vi "Maquina01Refrescos_1.vi"() -> ()   [LabVIEW 2018]
uses:
  EdoMaq1Refrescos.ctl
panel:
  in  "stop 2":bool
  out "Elapsed Time (s)":dbl
  out "Cambio":i32
  out "Suma":i32
  out "Edo":T1
  in  "stop":bool
  in  "Cancel Button":bool
  in  "$10":bool
  in  "$5":bool
  in  "$1":bool
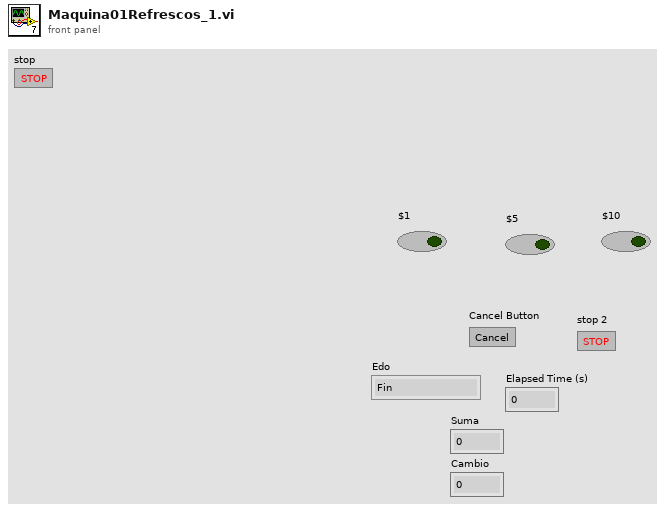
[diagram p1: front panel]
types:
  T1 = typedef "EdoMaq1Refrescos.ctl" = enum16{"Fin", "Espera", "JuntaDinero", "Entrega", "RegresaCambio", "Cancela"}
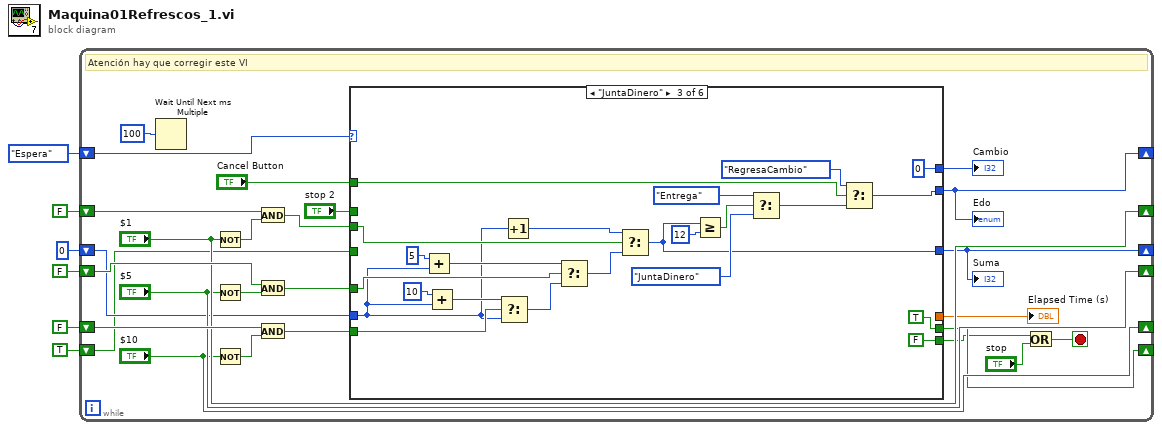
[diagram p0: block diagram]
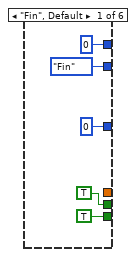
[diagram p2: hidden frame]
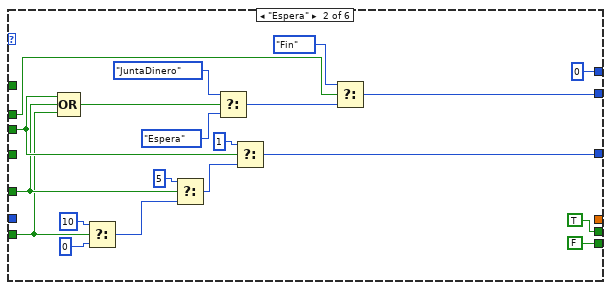
[diagram p3: hidden frame]
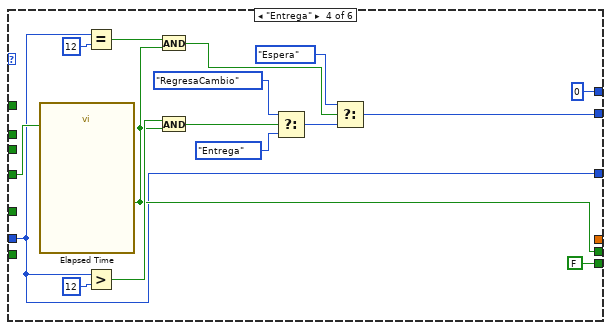
[diagram p4: hidden frame]
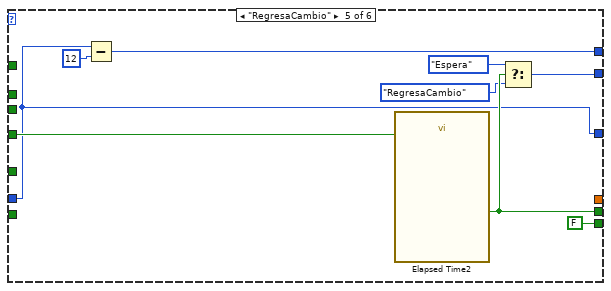
[diagram p5: hidden frame]
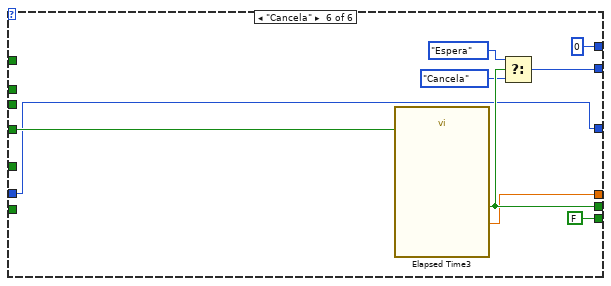
[diagram p6: hidden frame]
diagram:
  n1 = while {
    shift-right: [w17] -> _
    shift-left: EdoMaq1Refrescos."Espera" -> [w31]
    shift-right: ["$1"] -> _
    shift-left: FALSE -> [w29]
    shift-right: ["$5"] -> _
    shift-left: FALSE -> [w28]
    shift-right: ["$10"] -> _
    shift-left: FALSE -> [w27]
    shift-right: [w15] -> _
    shift-left: 0 -> [w16]
    shift-right: [w13] -> _
    shift-left: TRUE -> [w14]
    stop <- w8 stop-if-true
    # "Atención hay que corregir este VI"
    n2 = Wait Until Next ms Multiple(millisecond multiple=u32 100) -> ()  [unwired: 1 out]
    n3 = Not(x="$1") -> (.not. x?=w26:bool)
    n4 = Not(x="$5") -> (.not. x?=w25:bool)
    n5 = Not(x="$10") -> (.not. x?=w24:bool)
    n6 = And(x=w29, y=w26) -> (x .and. y?=w23:bool)
    n7 = And(x=w28, y=w25) -> (x .and. y?=w22:bool)
    n8 = And(x=w27, y=w24) -> (x .and. y?=w21:bool)
    n9 = case shown="\"JuntaDinero\"" w31 {
      tunnel: "Cancel Button" -> [_ _ w79 _ _ _]
      tunnel: w23 -> [_ w51 w77 _ _ _]
      tunnel: w22 -> [_ w48 w75 _ _ _]
      tunnel: w21 -> [_ w46 w72 _ _ _]
      tunnel: [EdoMaq1Refrescos."Fin" ("f") w53 w65 w84 w101 w110] -> w17
      tunnel: w16 -> [_ _ w58 w83 w98 w108]
      tunnel: [0 w38 w59 w83 w98 w108] -> w15
      tunnel: w14 -> [_ _ _ w96 w105 w114]
      tunnel: [TRUE ("Time has Elapsed") TRUE ("Time has Elapsed") TRUE ("Time has Elapsed") w88 w104 w113] -> w13
      tunnel: [0 0 0 0 w99 0] -> w12
      tunnel: [_ _ _ _ _ w107] -> w11
      tunnel: [TRUE FALSE FALSE FALSE FALSE FALSE] -> w9
      tunnel: "stop 2" -> [_ w39 _ _ _ _]
      frame "Fin", Default {
      }
      frame "Espera" {
        n10 = Compound Arithmetic op=OR(w51, w48, w46) -> (w54:bool)
        n11 = Select(t=10, s=w46, f=0) -> (s? t:f=w44:i32)
        n12 = Select(t=5, s=w48, f=w44) -> (s? t:f=w49:i32)
        n13 = Select(t=EdoMaq1Refrescos."JuntaDinero", s=w54, f=EdoMaq1Refrescos."Espera") -> (s? t:f=w57:T1)
        n14 = Select(t=1, s=w51, f=w49) -> (s? t:f=w38:i32)
        n15 = Select(t=EdoMaq1Refrescos."Fin", s=w39, f=w57) -> (s? t:f=w53:T1)
      }
      frame "JuntaDinero" {
        n16 = Add(x=5, y=w58) -> (x+y=w73:i32)
        n17 = Add(x=10, y=w58) -> (x+y=w70:i32)
        n18 = Select(t=w70, s=w72, f=w58) -> (s? t:f=w60:i32)
        n19 = Increment(x=w58) -> (x+1=w76:i32)
        n20 = Select(t=w73, s=w75, f=w60) -> (s? t:f=w61:i32)
        n21 = Select(t=w76, s=w77, f=w61) -> (s? t:f=w59:i32)
        n22 = Greater Or Equal?(x=w59, y=12) -> (x >= y?=w68:bool)
        n23 = Select(t=EdoMaq1Refrescos."Entrega", s=w68, f=EdoMaq1Refrescos."JuntaDinero") -> (s? t:f=w80:T1)
        n24 = Select(t=EdoMaq1Refrescos."RegresaCambio", s=w79, f=w80) -> (s? t:f=w65:T1)
      }
      frame "Entrega" {
        n25 = call "Elapsed Time"("Reset"=w96) -> ("Time has Elapsed"=w88:bool)  [unwired: 11 in, 7 out]
        n26 = Equal?(x=w83, y=12) -> (x = y?=w93:bool)
        n27 = Greater?(x=w83, y=12) -> (0:w89:bool)
        n28 = And(x=w93, y=w88) -> (x .and. y?=w92:bool)
        n29 = And(x=w89, y=w88) -> (x .and. y?=w87:bool)
        n30 = Select(t=EdoMaq1Refrescos."RegresaCambio", s=w87, f=EdoMaq1Refrescos."Entrega") -> (s? t:f=w95:T1)
        n31 = Select(t=EdoMaq1Refrescos."Espera", s=w92, f=w95) -> (s? t:f=w84:T1)
      }
      frame "RegresaCambio" {
        n32 = Subtract(x=w98, y=12) -> (x-y=w99:i32)
        n33 = call "Elapsed Time2"("Reset"=w105) -> ("Time has Elapsed"=w104:bool)  [unwired: 11 in, 7 out]
        n34 = Select(t=EdoMaq1Refrescos."Espera", s=w104, f=EdoMaq1Refrescos."RegresaCambio") -> (s? t:f=w101:T1)
      }
      frame "Cancela" {
        n35 = call "Elapsed Time3"("Reset"=w114) -> ("Elapsed Time (s)"=w107:dbl, "Time has Elapsed"=w113:bool)  [unwired: 11 in, 6 out]
        n36 = Select(t=EdoMaq1Refrescos."Espera", s=w113, f=EdoMaq1Refrescos."Cancela") -> (s? t:f=w110:T1)
      }
    }
    "Edo" <- w17
    "Suma" <- w15
    "Cambio" <- w12
    "Elapsed Time (s)" <- w11
    n37 = Or(x=w9, y="stop") -> (x .or. y?=w8:bool)
  }
